vi "CsTool-ErrorHandlerAll.vi"(1 "StopOnError (true)":bool=TRUE, 2 "Error Code":i32, 3 "Handle Cluster":T1) -> (0 "Error String":string)   [LabVIEW 2022 SP3]
doc: "This VI converts an error code, returned from a CsTool or CsLv VI, into a string that describes the error. Optionally, the VI can be configured to stop VI operation upon an error.\n\nIf the StopOnError flag is set to TRUE and the input error code indicates an error, the LabVIEW STOP function is called, which terminates VI operation. If StopOnError is set to FALSE, the error string is returned but VI execution will continue, if possible. The StopOnError default value is TRUE.\n\nIf the Handle Cluster is valid, the StopOnError input is set to TRUE, and the error code indicates an error, then CsTool-ErrorHandler.vi will free the specified CompuScope system so that it may be used by another program. The Handle Cluster uniquely identifies a CompuScope system and is obtained by using CsTool-GetSystem.vi."
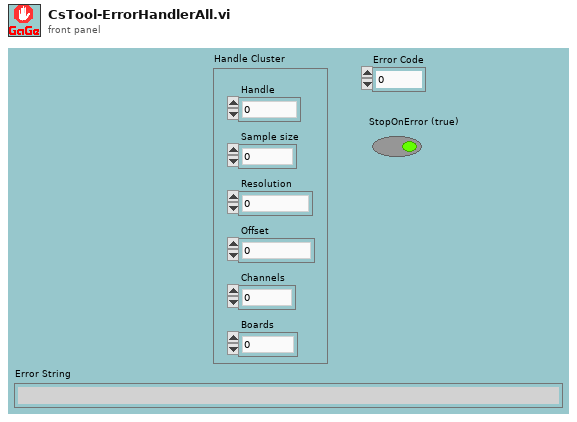
[diagram p1: front panel]
types:
  T1 = cluster{"Handle":u32, "Sample size":u32, "Resolution":i32, "Offset":i32, "Channels":u32, "Boards":u32}
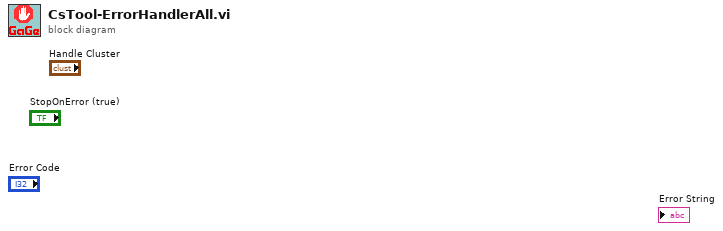
[diagram p0: block diagram]
diagram:
